vi "stC to K.vi"(8 "error in (no error)":errorcluster, 10 "stC (0)":dbl) -> (0 "error out":errorcluster, 2 "K":dbl)   [LabVIEW 2014]
doc: "Przelicza wartoœæ temperatury ze stopni celsjusza na Kelwiny"
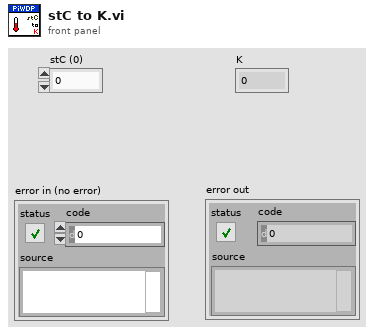
[diagram p1: front panel]
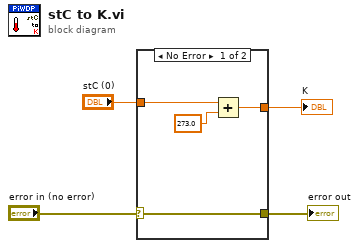
[diagram p0: block diagram]
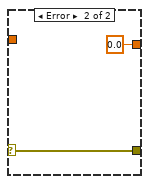
[diagram p2: hidden frame]
diagram:
  n1 = case shown="No Error" "error in (no error)" {
    selector: "error in (no error)" -> [w6 w9]
    tunnel: "stC (0)" -> [w8 _]
    tunnel: [w7 0.0] -> w3
    tunnel: [w6 w9] -> w1
    frame No Error {
      n2 = Add(x=w8, y=273.0) -> (x+y=w7:dbl)
    }
    frame Error {
    }
  }
  "K" <- w3
  "error out" <- w1
